vi "test_CCDGetChipSize.vi"(8 "error in":errorcluster) -> (0 "error out":errorcluster)   [LabVIEW 2023]
uses:
  Classes/CCD/CCD.lvclass
  C:/Projects/Horiba/horiba-labview-sdk/Source/Classes/GenericDevice/GenericDevice.lvclass
  <vilib>/addons/_JKI Toolkits/Caraya/classes/Assert/Assert Equal Value and Type_Variant.vi
  <vilib>/addons/_JKI Toolkits/Caraya/classes/Assert/Assert Not Error.vi
  <vilib>/addons/_JKI Toolkits/Caraya/classes/Test/Test.lvclass
  <vilib>/addons/_JKI Toolkits/Caraya/classes/Assert/Assert.lvclass
  C:/Projects/Horiba/horiba-labview-sdk/Source/Classes/CCD/CCD.lvclass
panel:
  # "Connector Pane"
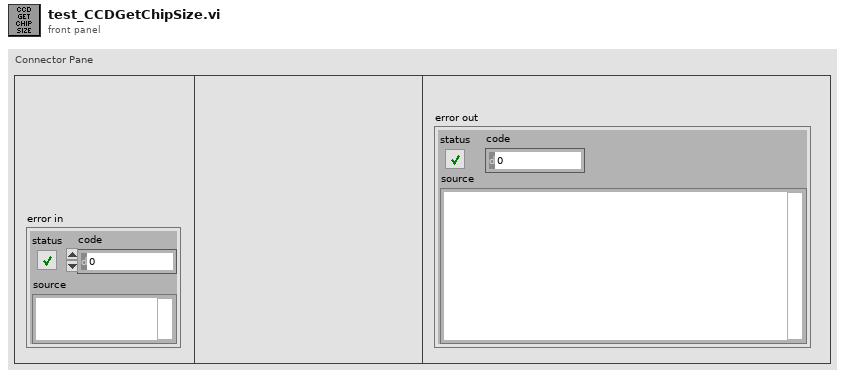
[diagram p1: front panel]
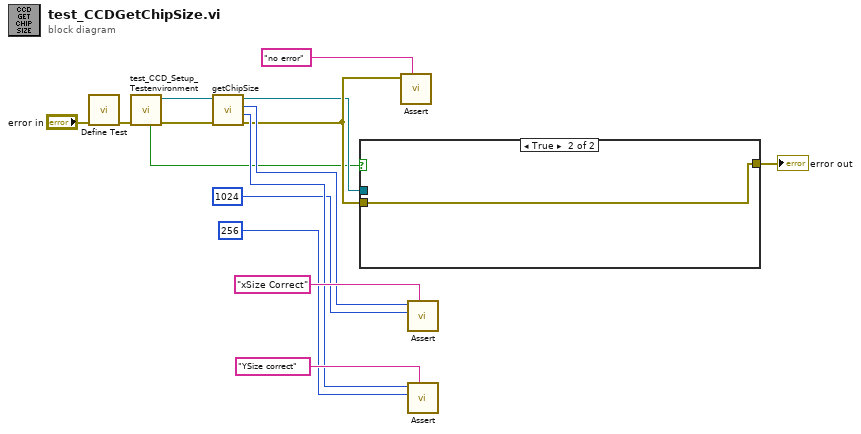
[diagram p0: block diagram]
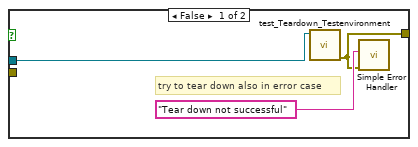
[diagram p2: hidden frame]
diagram:
  n1 = call <vilib>:"Define Test.vi"("error in (no error)"="error in") -> ("error out"=w3:errorcluster)  [unwired: 9 in, 1 out]
  n2 = call "test_CCD_Setup_Testenvironment.vi"("error in"=w3) -> ("error out"=w2:errorcluster, "CCD out"=w4:refnum<class "CCD.lvclass">, "Module Was Already Running?"=w1:bool)  [unwired: 7 in, 1 out]
  n3 = call-dynamic "getChipSize.vi"("error in (no error)"=w2, "CCD in"=w4) -> ("error out"=w7:errorcluster, "chip size, y"=w12:i32, "chip size, x"=w14:i32, "CCD out"=w6:refnum<class "CCD.lvclass">)  [unwired: 6 in]
  n4 = case shown="True" w1 {
    tunnel: w6 -> [w17 _]
    tunnel: [w16 w19] -> w5
    tunnel: w7 -> [_ w19]
    frame False {
      # "try to tear down also in error case"
      n5 = call "test_Teardown_Testenvironment.vi"("GenericDevice.lvclass"=w17) -> ("error out"=w16:errorcluster)  [unwired: 9 in, 1 out]
      n6 = call <vilib>:"Simple Error Handler.vi"("error source (\" \")"="Tear down not successful" ("error source (\" \")"), "error in (no error)"=w16) -> ()  [unwired: 3 in, 5 out]
    }
    frame True {
    }
  }
  "error out" <- w5
  n7 = call-poly <vilib>:"Assert.vi"("Label"="no error" ("Label (VI Title)"), "Not Error?"=w7) -> ()  [unwired: 8 in, 2 out]
  n8 = call-poly <vilib>:"Assert.vi"("Label"="xSize Correct" ("Label (VI Title)"), "Y"=1024, "X"=w14) -> ()  [unwired: 7 in, 2 out]
  n9 = call-poly <vilib>:"Assert.vi"("Label"="YSize correct" ("Label (VI Title)"), "Y"=256, "X"=w12) -> ()  [unwired: 7 in, 2 out]
